vi "AM Step CW.vi"(8 "error in (no error)":errorcluster, 10 "Message Queues in":T1, 11 "Data Cluster":T2 {"PS Measure Plan" items=["Pretreatment settings (PS)", "Linear Sweep Voltammetry (LSV)", "Differential Pulse Voltammetry (DPV)", "Cyclic Voltammetry (CV)", "Chronoamperometry (CA)", "Chronopotentiometry (CP)", "El Imp Spectroscopy (EIS)"]; "System Preset"."Test Configuration"."SP List" format="%#.1g"}) -> (0 "error out":errorcluster, 3 "Data Cluster out":T2 {"PS Measure Plan" items=["Pretreatment settings (PS)", "Linear Sweep Voltammetry (LSV)", "Differential Pulse Voltammetry (DPV)", "Cyclic Voltammetry (CV)", "Chronoamperometry (CA)", "Chronopotentiometry (CP)", "El Imp Spectroscopy (EIS)"]; "System Preset"."Test Configuration"."SP List" format="%#.1g"})   [LabVIEW 2020, in "Test Driver.lvlib"]
uses:
  Test Driver.lvlib
  Test Driver Configuration.ctl
  support/Message Queue/Message Cluster.ctl
  System Preset.ctl
  Test Type.ctl
  support/Message Queue/All Message Queues.ctl
  support/Message Queue/Message Queue.lvlib
panel:
  # "X"
  # "Y"
  # "Cycles"
  # "Point Delay"
  # "Up"
  # "Down"
  # "Z Axes"
  # "#C"
  # "In"
  # "Out"
  # "Cleaning [sec]"
  # "X"
  # "Y"
  # "Cycles"
  # "Point Delay"
  # "Up"
  # "Down"
  # "Z Axes"
  # "#C"
  # "In"
  # "Out"
  # "Cleaning [sec]"
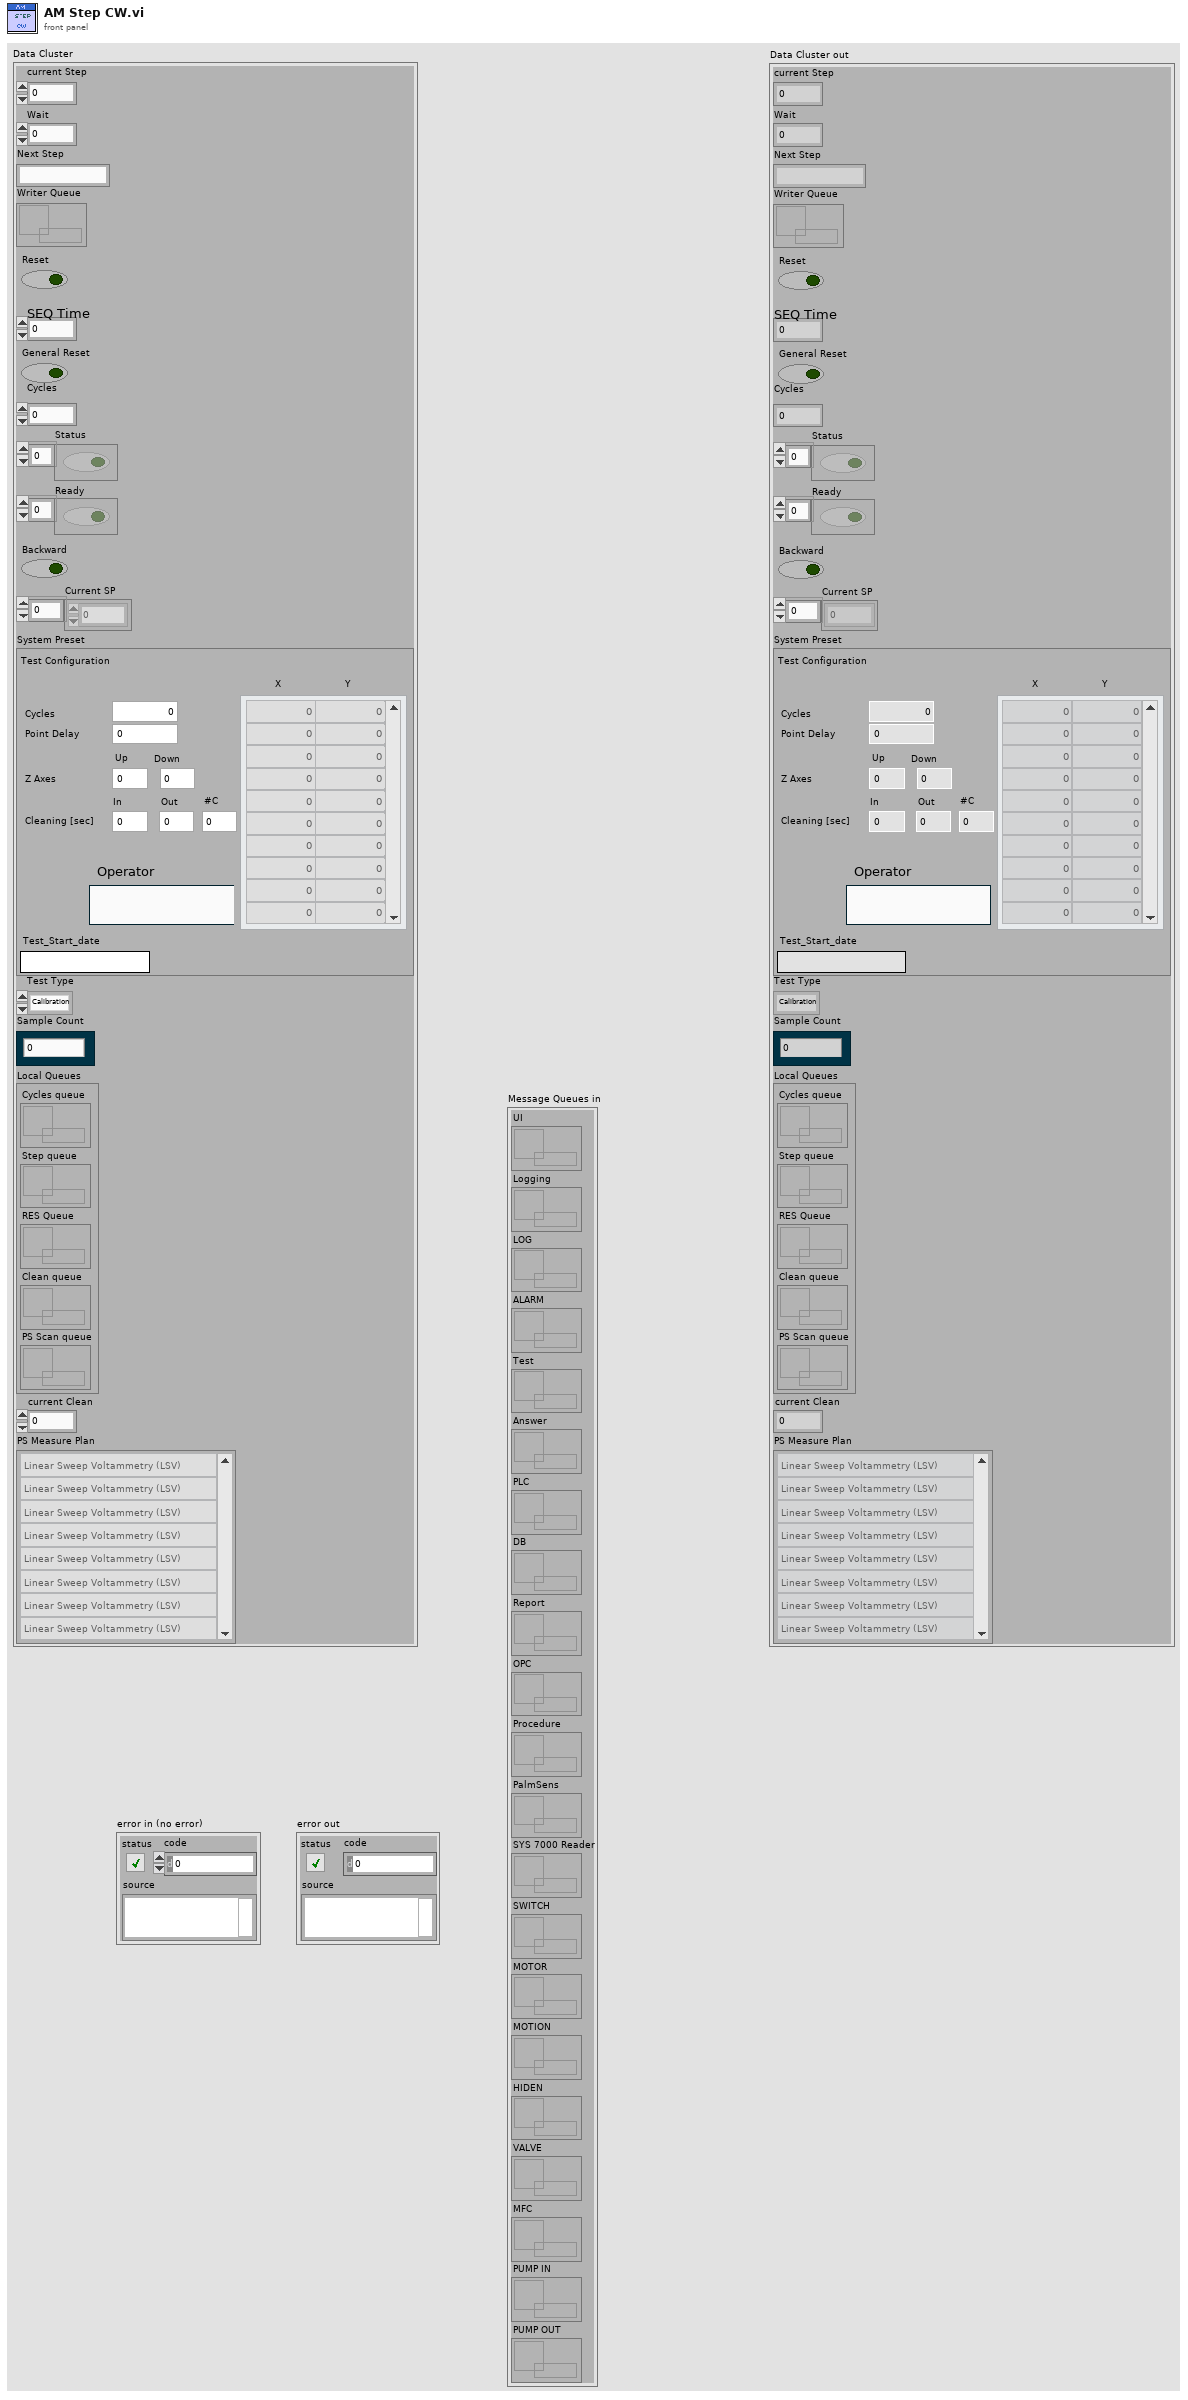
[diagram p1: front panel]
types:
  T1 = typedef "Message Queue.lvlib/All Message Queues.ctl" = cluster{"UI":refnum<queue>, "Logging":refnum<queue>, "LOG":refnum<queue>, "ALARM":refnum<queue>, "Test":refnum<queue>, "Answer":refnum<queue>, "PLC":refnum<queue>, "DB":refnum<queue>, "Report":refnum<queue>, "OPC":refnum<queue>, "Procedure":refnum<queue>, "PalmSens":refnum<queue>, "SYS 7000 Reader":refnum<queue>, "SWITCH":refnum<queue>, "MOTOR":refnum<queue>, "MOTION":refnum<queue>, "HIDEN":refnum<queue>, "VALVE":refnum<queue>, "MFC":refnum<queue>, "PUMP IN":refnum<queue>, "PUMP OUT":refnum<queue>}
  T2 = typedef "Test Driver.lvlib/Test Driver Configuration.ctl" = cluster{"current Step":i32, "Wait":dbl, "Next Step":string, "Writer Queue":refnum<queue>, "Reset":bool, "SEQ Time":i32, "General Reset":bool, "Cycles":i32, "Status":bool[], "Ready":bool[], "Backward":bool, "Current SP":dbl[], "System Preset":T3, "Test Type":T4, "Sample Count":i32, "Local Queues":cluster{"Cycles queue":refnum<queue>, "Step queue":refnum<queue>, "RES Queue":refnum<queue>, "Clean queue":refnum<queue>, "PS Scan queue":refnum<queue>}, "current Clean":i32, "PS Measure Plan":u16[]}
  T3 = typedef "System Preset.ctl" = cluster{"Test Configuration":cluster{"Cycles":i32, "Z Up":dbl, "SP List":dbl[][], "Operator":string, "Point Delay":i32, "Z Up 2":dbl, "Cleaning In":dbl, "Cleaning Out":dbl, "Cleaning Cycles":i32}, "Test_Start_date":string}
  T4 = typedef "Test Driver.lvlib/Test Type.ctl" = enum16{"Calibration", "Test"}
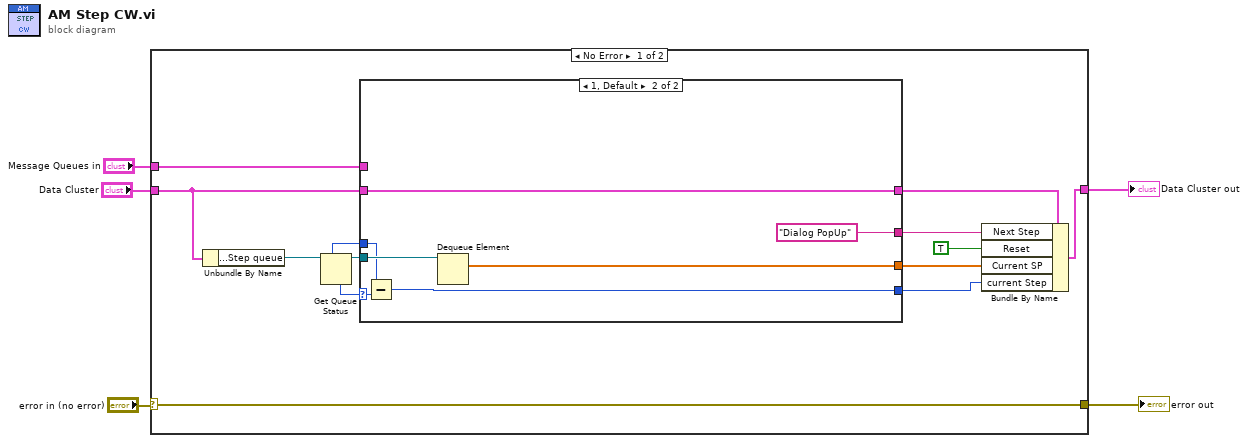
[diagram p0: block diagram]
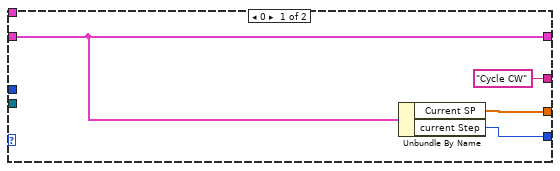
[diagram p2: hidden frame]
diagram:
  n1 = case shown="No Error" "error in (no error)" {
    selector: "error in (no error)" -> [w18 w30]
    tunnel: [w13 w31] -> w4
    tunnel: "Data Cluster" -> [w15 w31]
    tunnel: [w18 w30] -> w3
    tunnel: "Message Queues in" -> [w8 _]
    frame No Error {
      n2 = Unbundle By Name(w15) -> ("Local Queues.Step queue"=w17:refnum<queue>)
      n3 = Get Queue Status(queue=w17) -> (queue out=w16:refnum<queue>, max queue size=w9:i32, # elements in queue=w10:i32)  [unwired: 2 in, 5 out]
      n4 = case shown="1, Default" w10 {
        selector: w10 -> [_ w27]
        tunnel: w16 -> [_ w29]
        tunnel: [w21 w26] -> w14
        tunnel: w15 -> [w21 w26]
        tunnel: ["Cycle CW" "Dialog PopUp" ("Message")] -> w12
        tunnel: w8 -> [_ _]
        tunnel: w9 -> [_ w28]
        tunnel: [w20 w25] -> w7
        tunnel: [w19 w23] -> w6
        frame 0 {
          n5 = Unbundle By Name(w21) -> ("Current SP"=w20:dbl[], "current Step"=w19:i32)
        }
        frame 1, Default {
          n6 = Subtract(x=w28, y=w27) -> (x-y=w23:i32)
          n7 = Dequeue Element(queue=w29) -> (element=w25:dbl[])  [unwired: 2 in, 3 out]
        }
      }
      n8 = Bundle By Name(cluster=w14, "Next Step"=w12, "Reset"=TRUE, "Current SP"=w7, "current Step"=w6) -> (w13:T2)
    }
    frame Error {
    }
  }
  "error out" <- w3
  "Data Cluster out" <- w4
